vi "Rollendrehzahl (SubVI).vi"(7 "dT(Rolle) (Eingang)":refnum<vi>, 8 "Cyclecounter":refnum<vi>, 9 "Stop":refnum<vi>, 10 "Rollendrehzahl aufzeichnen":refnum<vi>, 11 "n(Rolle) (Eingang)":refnum<vi>) -> ()   [LabVIEW 2014]
panel:
  in  "Export":bool
  in  "Reset Graph":bool
  in  "Aufzeichnung":bool
  out "Rollendrehzahl":cluster{dbl[], dbl[]}(graph)
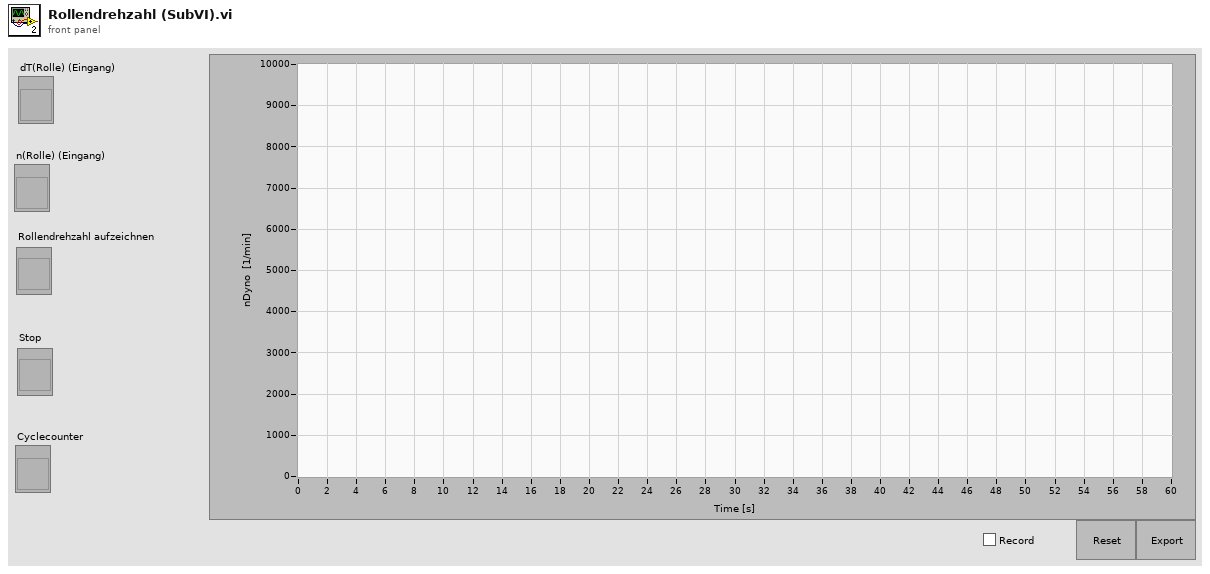
[diagram p1: front panel]
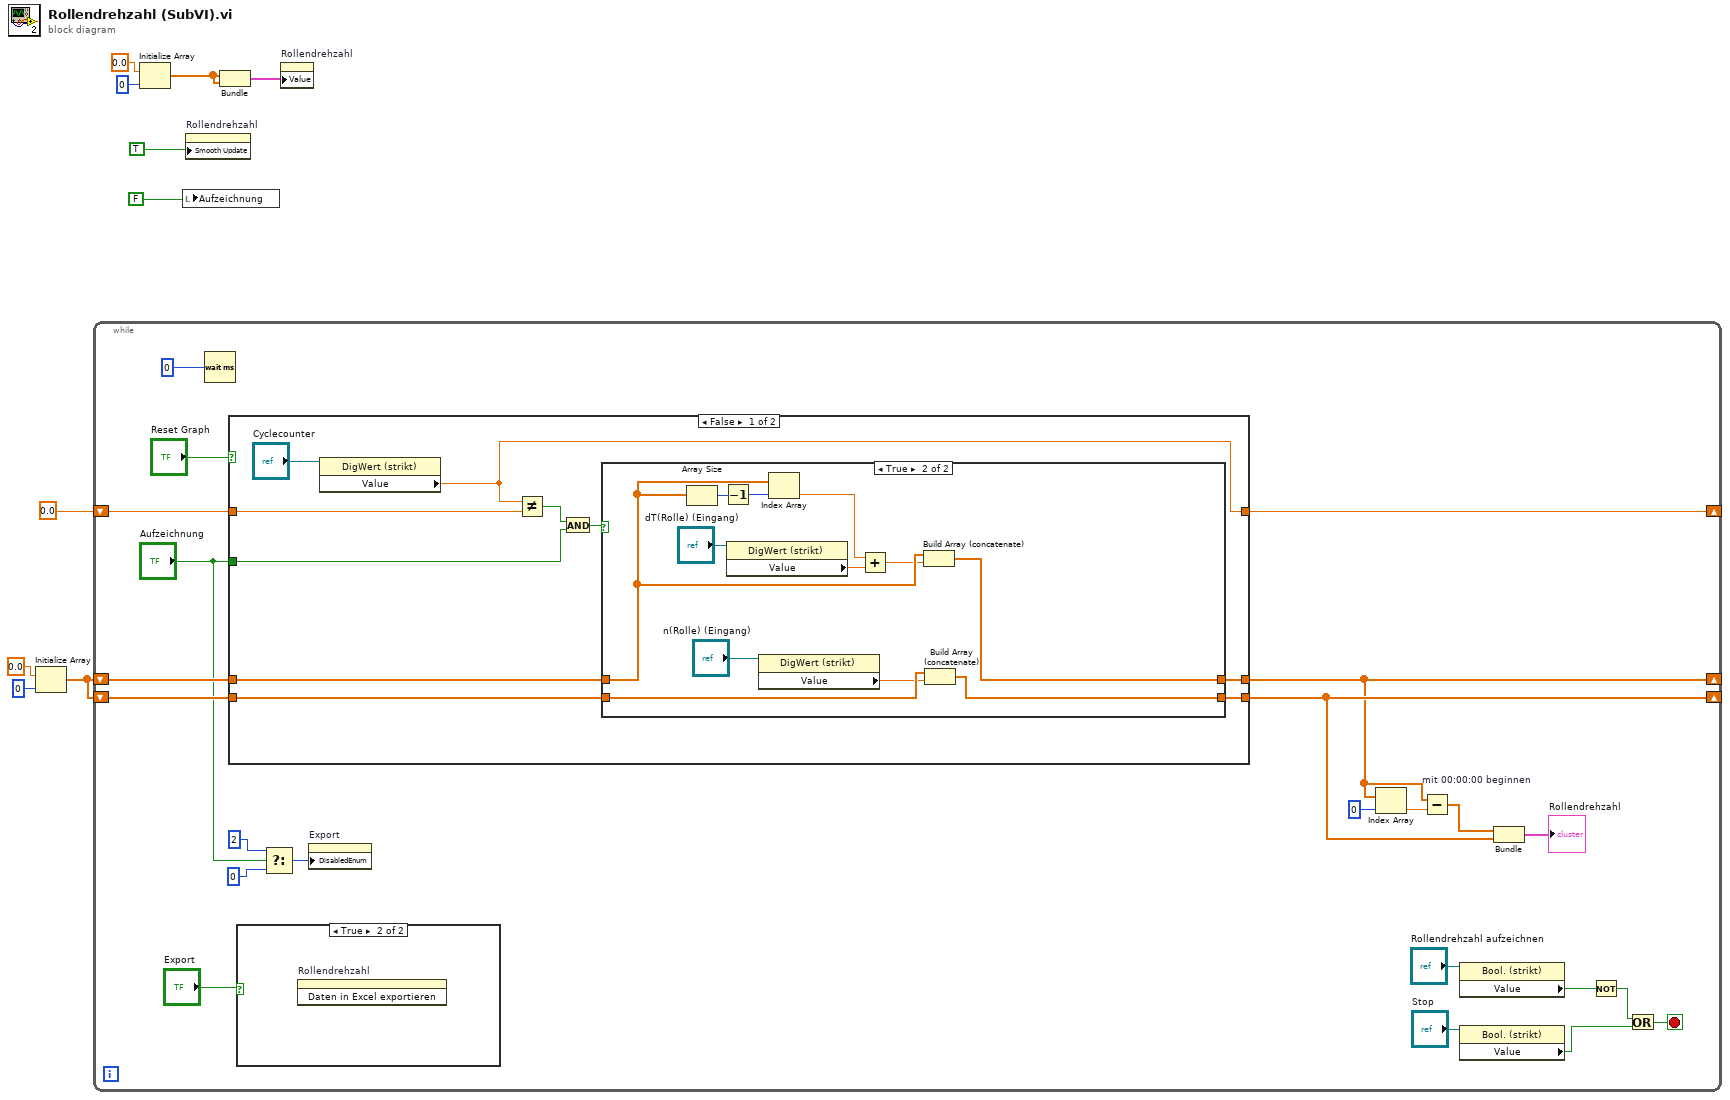
[diagram p0: block diagram]
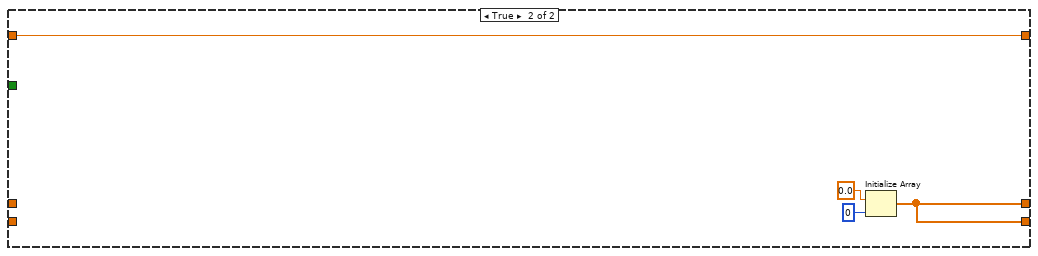
[diagram p4: hidden frame]
diagram:
  n1 = Initialize Array(0.0 ("y"), 0) -> (w7:dbl[])
  n2 = while {
    shift-right: [w16] -> _
    shift-left: w7 -> [w31]
    shift-right: [w12] -> _
    shift-left: w7 -> [w24]
    shift-right: [w22] -> _
    shift-left: 0.0 -> [w23]
    stop <- w28 stop-if-true
    n3 = Wait (ms)(milliseconds to wait=0) -> ()  [unwired: 1 out]
    n4 = case shown="False" "Reset Graph" {
      tunnel: w31 -> [w43 _]
      tunnel: [w42 w59] -> w16
      tunnel: w24 -> [w41 _]
      tunnel: [w40 w59] -> w12
      tunnel: w23 -> [w39 w58]
      tunnel: [w35 w58] -> w22
      tunnel: "Aufzeichnung" -> [w34 _]
      frame False {
        n5 = property class="DigWert (strikt)"(reference="Cyclecounter") -> ("Value"=w35:dbl)  [unwired: 1 in, 2 out]
        n6 = Not Equal?(x=w35, y=w39) -> (x != y?=w37:bool)
        n7 = And(x=w37, y=w34) -> (x .and. y?=w38:bool)
        n8 = case shown="True" w38 {
          tunnel: w43 -> [w45 w57]
          tunnel: [w45 w56] -> w42
          tunnel: w41 -> [w44 w55]
          tunnel: [w44 w46] -> w40
          frame False {
          }
          frame True {
            n9 = Array Size(array=w55) -> (size(s)=w52:i32)
            n10 = Decrement(x=w52) -> (x-1=w51:i32)
            n11 = property class="DigWert (strikt)"(reference="dT(Rolle) (Eingang)") -> ("Value"=w48:dbl)  [unwired: 1 in, 2 out]
            n12 = property class="DigWert (strikt)"(reference="n(Rolle) (Eingang)") -> ("Value"=w54:dbl)  [unwired: 1 in, 2 out]
            n13 = Index Array(array=w55, index=w51) -> (element=w49:dbl)
            n14 = Add(x=w49, y=w48) -> (x+y=w47:dbl)
            n15 = Build Array (concatenate)(w55, w47) -> (w46:dbl[])
            n16 = Build Array (concatenate)(w57, w54) -> (w56:dbl[])
          }
        }
      }
      frame True {
        n17 = Initialize Array(0.0 ("y"), 0) -> (w59:dbl[])
      }
    }
    n18 = case shown="True" "Export" {
      frame False {
      }
      frame True {
        n19 = invoke on="Rollendrehzahl" class="XYGraph (strikt)" method="Daten in Excel exportieren"() -> ()  [unwired: 3 in, 3 out]
      }
    }
    n20 = Select(t=2, s="Aufzeichnung", f=0) -> (s? t:f=w20:i32)
    n21 = property on="Export" class="Bool."("DisabledEnum"=w20) -> ()  [unwired: 2 in, 2 out]
    n22 = Index Array(array=w12, index=0) -> (element=w15:dbl)
    n23 = Subtract "mit 00:00:00 beginnen"(x=w12, y=w15) -> (x-y=w13:dbl[])
    n24 = property class="Bool. (strikt)"(reference="Rollendrehzahl aufzeichnen") -> ("Value"=w32:bool)  [unwired: 1 in, 2 out]
    n25 = property class="Bool. (strikt)"(reference="Stop") -> ("Value"=w25:bool)  [unwired: 1 in, 2 out]
    n26 = Bundle(w13, w16) -> (→"Rollendrehzahl":cluster{dbl[], dbl[]})  [unwired: 1 in]
    n27 = Not(x=w32) -> (.not. x?=w26:bool)
    n28 = Or(x=w26, y=w25) -> (x .or. y?=w28:bool)
  }
  n29 = Initialize Array(0.0 ("y"), 0) -> (w2:dbl[])
  n30 = local write "Aufzeichnung"(FALSE) -> ()
  n31 = property on="Rollendrehzahl" class="XYGraph (strikt)"("Smooth Update"=TRUE) -> ()  [unwired: 2 in, 2 out]
  n32 = Bundle(w2, w2) -> (w5:cluster{dbl[], dbl[]})  [unwired: 1 in]
  n33 = property on="Rollendrehzahl" class="XYGraph (strikt)"("Value"=w5) -> ()  [unwired: 2 in, 2 out]
